vi "ParseOneTypeVariablesLine.vi"(0 "spreadsheet string":string) -> (1 "Input varables type":string[](array[string]), 2 "Input varables names":string[](array[string]), 3 "Input varables ports":i32[](array[numeric]), 4 "Input varables bytes":i32[](array[numeric]))   [LabVIEW 2012]
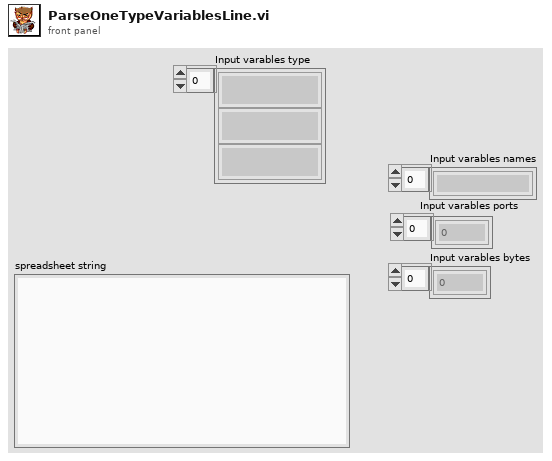
[diagram p1: front panel]
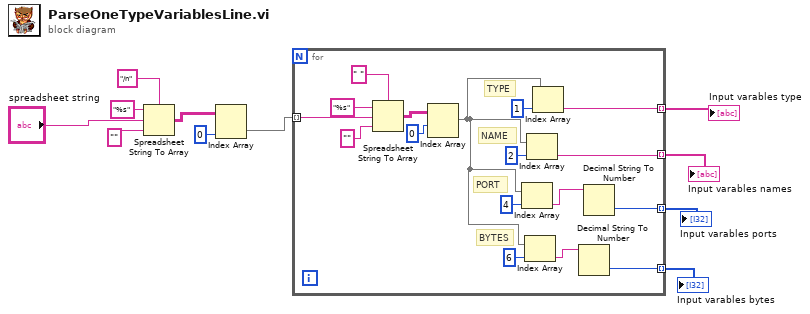
[diagram p0: block diagram]
diagram:
  n1 = Spreadsheet String To Array(delimiter (Tab)="/n", format string="%s", spreadsheet string="spreadsheet string", array type (2D Dbl)="" ("delimiter (Tab)")) -> (array=w8:string[][])
  n2 = Index Array(array=w8, index (col)=0 ("disabled index (col)")) -> (element=w7:string[])  [unwired: 1 in]
  n3 = for {
    tunnel: w7 -> [w27] mode=indexing
    tunnel: [w16] -> w4 mode=indexing
    tunnel: [w15] -> w3 mode=indexing
    tunnel: [w14] -> w2 mode=indexing
    tunnel: [w13] -> w1 mode=indexing
    # "BYTES"
    # "PORT"
    # "NAME"
    # "TYPE"
    n4 = Spreadsheet String To Array(delimiter (Tab)=" ", format string="%s", spreadsheet string=w27, array type (2D Dbl)="" ("delimiter (Tab)")) -> (array=w25:string[][])
    n5 = Index Array(array=w25, index (row)=0 ("disabled index (col)")) -> (element=w19:string[])  [unwired: 1 in]
    n6 = Index Array(array=w19, index=4) -> (element=w18:string)
    n7 = Index Array(array=w19, index=6) -> (element=w17:string)
    n8 = Index Array(array=w19, index=2) -> (element=w15:string)
    n9 = Index Array(array=w19, index=1) -> (element=w16:string)
    n10 = Decimal String To Number(string=w17) -> (number=w13:i32)  [unwired: 2 in, 1 out]
    n11 = Decimal String To Number(string=w18) -> (number=w14:i32)  [unwired: 2 in, 1 out]
  }
  "Input varables type" <- w4
  "Input varables names" <- w3
  "Input varables ports" <- w2
  "Input varables bytes" <- w1
